vi "Overline Cross.vi"(5 "Color":u32(colorbox), 7 "error in (no error)":errorcluster, 8 "Overlay Group":string, 9 "point":cluster{"x":i16, "y":i16}, 10 "Image In":T1) -> (0 "error out":errorcluster, 3 "Image Out":T1)   [LabVIEW 2009, in "POLARIS IMAQ Display.xctl"]
uses:
  POLARIS IMAQ Display.xctl
  <vilib>/vision/Image Controls.llb/IMAQ Image.ctl
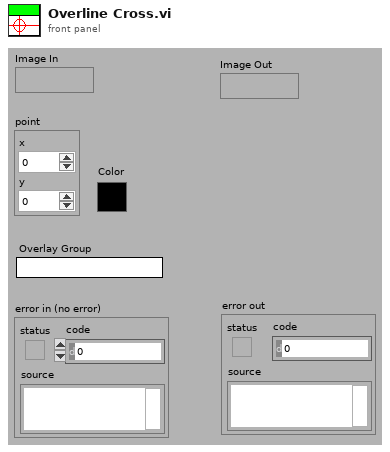
[diagram p1: front panel]
types:
  T1 = typedef "IMAQ Image.ctl" = refnum<image>
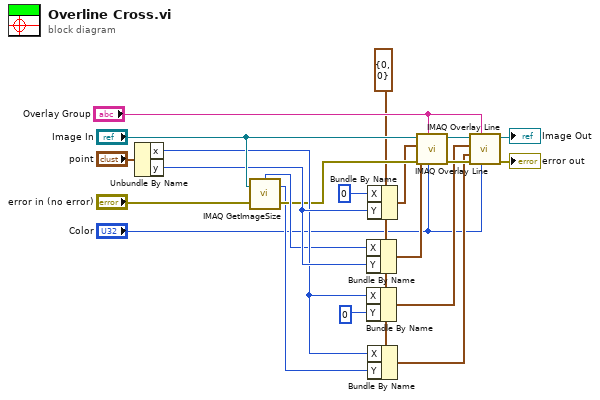
[diagram p0: block diagram]
diagram:
  w8 = cluster{"X":i32, "Y":i32} {"X"=0, "Y"=0} ("Start Point")
  n1 = Unbundle By Name("point") -> ("x"=w14:i16, "y"=w15:i16)
  n2 = call "IMAQ GetImageSize"("Image"="Image In", "error in (no error)"="error in (no error)") -> ("Y Resolution"=w11:i32, "X Resolution"=w13:i32, "error out"=w12:errorcluster)  [unwired: 2 in]
  n3 = Bundle By Name(cluster=w8, "X"=w13, "Y"=w15) -> (w6:cluster{"X":i32, "Y":i32})
  n4 = Bundle By Name(cluster=w8, "X"=w14, "Y"=0) -> (w3:cluster{"X":i32, "Y":i32})
  n5 = Bundle By Name(cluster=w8, "X"=0 ("Y"), "Y"=w15) -> (w7:cluster{"X":i32, "Y":i32})
  n6 = Bundle By Name(cluster=w8, "X"=w14, "Y"=w11) -> (w2:cluster{"X":i32, "Y":i32})
  n7 = call "IMAQ Overlay Line"("Color"="Color", "Group"="Overlay Group", "error in (no error)"=w12, "End Point"=w6, "Start Point"=w7, "Image"="Image In") -> ("error out"=w9:errorcluster, "Image Out"=w10:T1)  [unwired: 4 in]
  n8 = call "IMAQ Overlay Line"("Color"="Color", "Group"="Overlay Group", "error in (no error)"=w9, "End Point"=w2, "Start Point"=w3, "Image"=w10) -> ("error out"=→"error out":errorcluster, "Image Out"=→"Image Out":T1)  [unwired: 4 in]
